vi "CyberSim.vi"() -> ()   [LabVIEW 2013]
doc: "Top-level VI to run one simulation of the iRobot and environment."
uses:
  CyberSim interface/Simulation Configuration.ctl
  autograder/feedbackMode.ctl
  shared/iRobot Sensor Display.ctl
  iRobot/Sensor/Accelerometer.ctl
panel:
  in  "check grade":bool
  out "sequence number":i32
  in  "home camera":bool
  in  "play":bool
  out "Simulator Display":refnum<vi>(3d-picture)
  out "simulation running":bool
  in  "exit":bool
  in  "start":bool
  in  "stop":bool
  in  "pause":bool
  out "iRobot Sensor Display":T1 {"Right Wheel (mm/s)" scale=-500.0..500.0; "Left Wheel (mm/s)" scale=-500.0..500.0}
  in  "Front Panel Tabs":T3(tab)=enum."Configuration"
  out "Statechart Diagram Display (supports LabVIEW Statecharts only)":picture
  out "Feedback":string
  in  "simulation configuration":T4={"maxTime"=inf, "enableVisualization"=TRUE, "statechart"=path "../src/LabVIEW/Statechart/Simulation Statechart.vi", "environment"=path "Environment - Navigation and Hill Climb 1.xml", "record"=path "Simulation Record.xml", "autograde?"=FALSE, "interactive?"=FALSE, "feedback mode"=enum."debug navigation"}
  in  "save configuration":bool
  in  "terminate at simulation end?":bool
  out "simulation time (s)":sgl format="%7.3g"
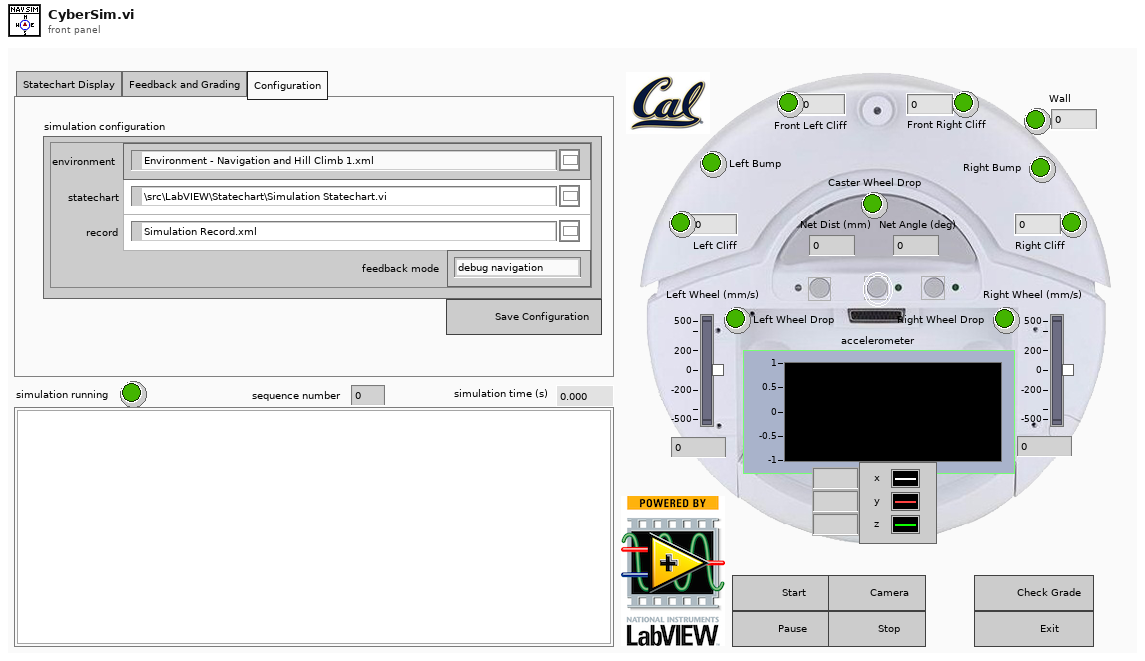
[diagram p1: front panel]
types:
  T1 = typedef "iRobot Sensor Display.ctl" = cluster{"Caster Wheel Drop":bool, "Left Wheel Drop":bool, "Right Wheel Drop":bool, "Left Bump":bool, "Right Bump":bool, "Left Cliff":bool, "Front Left Cliff":bool, "Front Right Cliff":bool, "Right Cliff":bool, "Wall":bool, "Net Dist (mm)":i32, "Net Angle (deg)":i32, "Wall":u16, "Left Cliff":u16, "Front Left Cliff":u16, "Front Right Cliff":u16, "Right Cliff":u16, "Left Wheel (mm/s)":i16, "Right Wheel (mm/s)":i16, "accelerometer":T2}
  T2 = typedef "Accelerometer.ctl" = cluster{"x axis (g)":dbl, "y axis (g)":dbl, "z axis (g)":dbl}
  T3 = enum32{"Statechart Display", "Feedback and Grading", "Configuration"}
  T4 = typedef "Simulation Configuration.ctl" = cluster{"maxTime":sgl, "enableVisualization":bool, "statechart":path, "environment":path, "record":path, "autograde?":bool, "interactive?":bool, "feedback mode":T5}
  T5 = typedef "feedbackMode.ctl" = enum32{"debug navigation", "debug hill climb", "autograde navigation", "autograde hill climb"}
  T6 = typedef "Simulator.ctl" = cluster{"configuration":T4, "Bump Sensors":refnum<k20>[], "Distance Sensors":refnum<k20>[], "Accelerometer":refnum<k20>, "Wall Sensor":refnum<k20>, "Statechart\ndisplay":refnum<vi>, "Body":refnum<k20>, "Left Motor":refnum<class "DC Motor Controller.lvclass">, "Right Motor":refnum<class "DC Motor Controller.lvclass">, "first step?":bool}
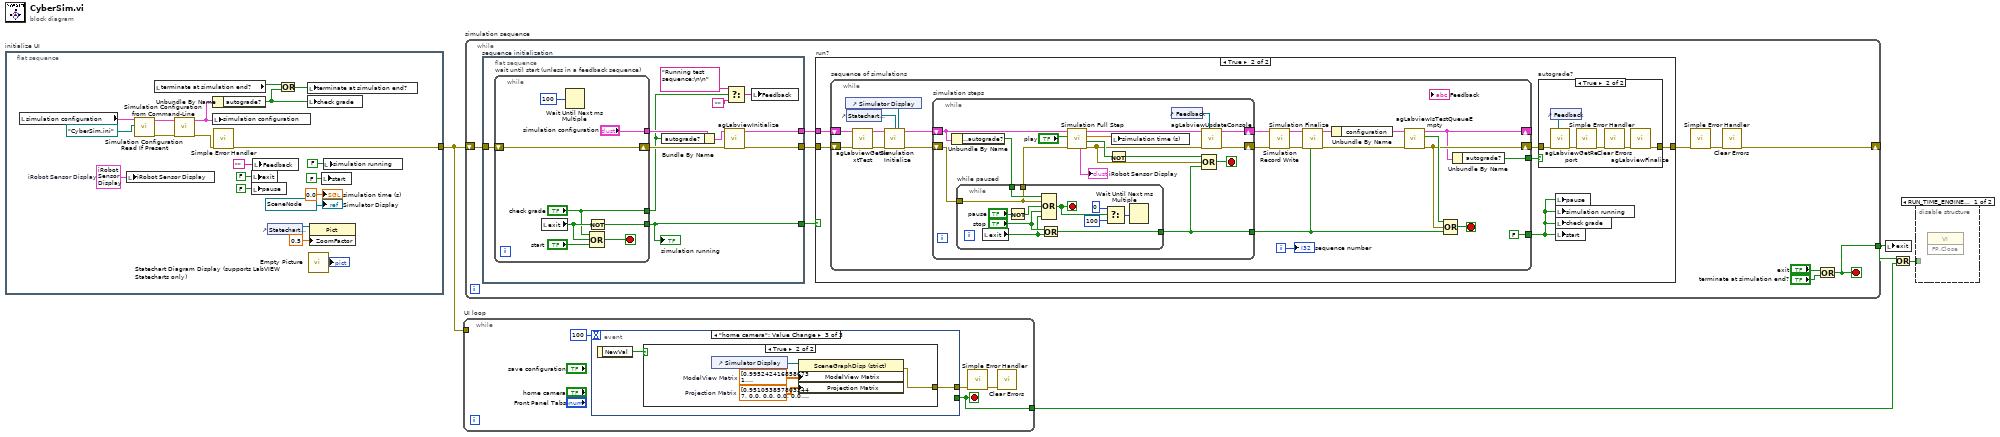
[diagram p0: block diagram]
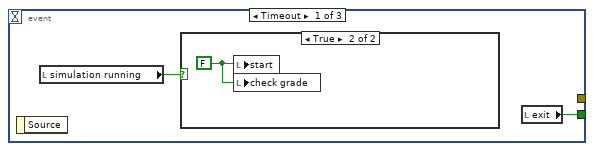
[diagram p3: hidden frame]
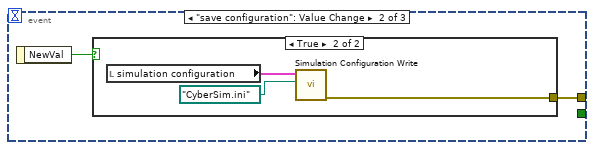
[diagram p5: hidden frame]
diagram:
  n1 = flat-sequence "initialize UI" {
    tunnel: [w21] -> w4
    frame #0 {
      w24 = T1 {"Caster Wheel Drop"=FALSE, "Left Wheel Drop"=FALSE, "Right Wheel Drop"=FALSE, "Left Bump"=FALSE, "Right Bump"=FALSE, "Left Cliff"=FALSE, "Front Left Cliff"=FALSE, "Front Right Cliff"=FALSE, "Right Cliff"=FALSE, "Wall"=FALSE, "Net Dist (mm)"=0, "Net Angle (deg)"=0, "Wall"=0, "Left Cliff"=0, "Front Left Cliff"=0, "Front Right Cliff"=0, "Right Cliff"=0, "Left Wheel (mm/s)"=0, "Right Wheel (mm/s)"=0, "accelerometer"={"x axis (g)"=0.0, "y axis (g)"=0.0, "z axis (g)"=0.0}}  # iRobot Sensor Display
      n2 = local read "simulation configuration"() -> (w19:T4)
      n3 = local write "iRobot Sensor Display"(w24) -> ()
      n4 = call "Simulation Configuration Read If Present.vi"("configuration"=path "CyberSim.ini", "simulation configuration"=w19) -> ("error out"=w17:errorcluster, "simulation configuration"=w18:T4)  [unwired: 8 in]
      n5 = local read "terminate at simulation end?"() -> (w9:bool)
      n6 = call "Simulation Configuration from Command-Line.vi"("error in"=w17, "simulation configuration in"=w18) -> ("error out"=w16:errorcluster, "simulation configuration out"=w14:T4)  [unwired: 8 in]
      n7 = Unbundle By Name(w14) -> ("autograde?"=w8:bool)
      n8 = local write "simulation configuration"(w14) -> ()
      n9 = call <vilib>:"Simple Error Handler.vi"("error in (no error)"=w16) -> ("error out"=w21:errorcluster)  [unwired: 4 in, 4 out]
      n10 = local write "exit"(FALSE ("exit")) -> ()
      n11 = local write "pause"(FALSE ("pause")) -> ()
      n12 = local write "Feedback"("") -> ()
      n13 = control-ref of="Statechart Diagram Display (supports LabVIEW Statecharts only)"() -> (w6:refnum<vi>)
      n14 = Or(x=w9, y=w8) -> (x .or. y?=w10:bool)
      n15 = local write "terminate at simulation end?"(w10) -> ()
      n16 = local write "check grade"(w8) -> ()
      n17 = call "Empty Picture"() -> ("empty picture"=→"Statechart Diagram Display (supports LabVIEW Statecharts only)":picture)
      n18 = property class="Pict"(reference=w6, "ZoomFactor"=sgl 0.5 ("Zoom Factor")) -> ()  [unwired: 1 in, 2 out]
      n19 = local write "start"(FALSE ("start")) -> ()
      n20 = local write "simulation running"(FALSE ("simulation running")) -> ()
      "simulation time (s)" <- sgl 0.0 ("simulated time (s)")
      "Simulator Display" <- refnum<vi> refnum ("3D Picture")
    }
  }
  n21 = while "UI loop" {
    tunnel: [w27] -> w2
    tunnel: w4 -> [_]
    stop <- w27 stop-if-true
    n22 = event shown="[2] \"home camera\": Value Change" {
      selector: _ -> [_ _ _]
      dyn-events: _ -> [_ _ _]
      timeout: 100 -> [_ _ _]
      tunnel: [_ w33 w38] -> w28
      tunnel: [w31 _ _] -> w27
      event Timeout {
        n23 = event-data() -> ()  [unwired: 1 in, 1 out]
        n24 = local read "simulation running"() -> (w30:bool)
        n25 = case shown="True" w30 {
          frame False {
          }
          frame True {
            w32 = FALSE ("AutoGrade")
            n26 = local write "start"(w32) -> ()
            n27 = local write "check grade"(w32) -> ()
          }
        }
        n28 = local read "exit"() -> (w31:bool)
      }
      event "save configuration": Value Change {
        n29 = event-data() -> ("NewVal"=w34:bool)  [unwired: 1 in]
        n30 = case shown="True" w34 {
          tunnel: [_ w36] -> w33
          frame False {
          }
          frame True {
            n31 = local read "simulation configuration"() -> (w37:T4)
            n32 = call "Simulation Configuration Write.vi"("configuration"=path "CyberSim.ini", "simulation configuration"=w37) -> ("error out"=w36:errorcluster)  [unwired: 9 in]
          }
        }
      }
      event "home camera": Value Change {
        n33 = event-data() -> ("NewVal"=w39:bool)  [unwired: 1 in]
        n34 = case shown="True" w39 {
          tunnel: [_ w40] -> w38
          frame False {
          }
          frame True {
            w41 = sgl[][] [[0.95105386, 0.0, 0.0, 0.0], [0.0, 2.4142137, 0.0, 0.0], [0.0, 0.0, -1.0002, -0.020002], [0.0, 0.0, -1.0, 0.0]]  # Projection Matrix
            w42 = sgl[][] [[0.9952424, -0.09162651, 0.033122927, -2.4552457], [0.010721975, 0.44090375, 0.8974903, -1.0543748], [-0.09683793, -0.8928653, 0.43978852, -0.9396557], [0.0, 0.0, 0.0, 1.0]]  # ModelView Matrix
            n35 = control-ref of="Simulator Display"() -> (w43:refnum<vi>)
            n36 = property class="SceneGraphDisp (strict)"(reference=w43, "ModelView Matrix"=w42, "Projection Matrix"=w41) -> (error out=w40:errorcluster)  [unwired: 1 in, 1 out]
          }
        }
      }
    }
    n37 = call <vilib>:"Simple Error Handler.vi"("error in (no error)"=w28) -> ("error out"=w26:errorcluster)  [unwired: 4 in, 4 out]
    n38 = call <vilib>:"Clear Errors.vi"("error in (no error)"=w26) -> ()  [unwired: 6 in, 1 out]
  }
  n39 = while "simulation sequence" {
    tunnel: [w50] -> w3
    shift-right: [w48] -> _
    shift-left: w4 -> [w44]
    stop <- w50 stop-if-true
    n40 = flat-sequence "sequence initialization" {
      tunnel: [w126] -> w49
      tunnel: [w127] -> w47
      tunnel: [w122] -> w46
      tunnel: w44 -> [w125]
      frame #0 {
        n41 = while "wait until start (unless in a feedback sequence)" {
          shift-right: [w132] -> w124
          shift-left: w125 -> [w132]
          tunnel: ["check grade"] -> w121
          tunnel: ["simulation configuration"] -> w123
          tunnel: [w129] -> w122
          stop <- w136 stop-if-true
          n42 = local read "exit"() -> (w135:bool)
          n43 = Wait Until Next ms Multiple(millisecond multiple=u32 100) -> ()  [unwired: 1 out]
          n44 = Not(x=w135) -> (.not. x?=w129:bool)
          n45 = Compound Arithmetic op=OR("check grade", w135, "start") -> (w136:bool)
        }
        "simulation running" <- w122
        n46 = Bundle By Name(cluster=w123, "autograde?"=w121) -> (w128:T4)
        n47 = call "agLabviewInitialize.vi"("Error In"=w124, "simulation configuration"=w128) -> ("Error Out"=w127:errorcluster, "simulation configuration"=w126:T4)  [unwired: 8 in]
        n48 = Select(t="Running test sequence:\n\n", s=w121, f="") -> (s? t:f=w119:string)
        n49 = local write "Feedback"(w119) -> ()
      }
    }
    n50 = case "run?" shown="True" w46 {
      tunnel: w49 -> [_ w60]
      tunnel: w47 -> [w54 w59]
      tunnel: [w54 w56] -> w45
      frame False {
      }
      frame True {
        n51 = while "sequence of simulations" {
          shift-right: [w78] -> w57
          shift-left: w59 -> [w73]
          shift-right: [w68] -> _
          shift-left: w60 -> [w72]
          tunnel: [w77] -> w58
          tunnel: [FALSE] -> w55
          i -> [w90]
          stop <- w89 stop-if-true
          n52 = control-ref of="Simulator Display"() -> (w84:refnum<vi>)
          n53 = control-ref of="Statechart Diagram Display (supports LabVIEW Statecharts only)"() -> (w86:refnum<vi>)
          n54 = call "agLabviewGetNextTest.vi"("Error In"=w73, "simulation configuration"=w72) -> ("Error Out"=w74:errorcluster, "simulation configuration"=w75:T4)  [unwired: 8 in]
          n55 = call "Simulation Initialize.vi"("simulation configuration"=w75, "Statechart display"=w86, "Simulator display"=w84, "Error In"=w74) -> ("simulator"=w88:T6, "Error Out"=w87:errorcluster)  [unwired: 10 in]
          n56 = while "simulation steps" {
            shift-right: [w93] -> w83
            shift-left: w88 -> [w99]
            shift-right: [w92] -> w85
            shift-left: w87 -> [w97]
            tunnel: [w100] -> w79
            stop <- w104 stop-if-true
            n57 = Unbundle By Name(w99) -> ("configuration.autograde?"=w98:bool)
            n58 = while "while paused" {
              tunnel: [w113] -> w100
              tunnel: w97 -> [w107]
              tunnel: w98 -> [w108]
              tunnel: [w107] -> w96
              stop <- w109 stop-if-true
              n59 = local read "exit"() -> (w114:bool)
              n60 = Not(x="pause") -> (.not. x?=w116:bool)
              n61 = Or(x="stop", y=w114) -> (x .or. y?=w113:bool)
              n62 = Compound Arithmetic op=OR(w108, w107, w116, "stop", w114) -> (w109:bool)
              n63 = Select(t=u32 0 ("millisecond multiple"), s=w109, f=u32 100 ("millisecond multiple")) -> (s? t:f=w112:u32)
              n64 = Wait Until Next ms Multiple(millisecond multiple=w112) -> ()  [unwired: 1 out]
            }
            n65 = call "Simulation Full Step.vi"("Error In"=w96, "iRobot Play Button (false)"="play", "simulator"=w99) -> ("Error Out"=w95:errorcluster, "continue to next step?"=w105:bool, "simulated time (s)"=w102:sgl, "simulator"=w94:T6, "iRobot Sensor Display"=→"iRobot Sensor Display":T1)  [unwired: 4 in]
            n66 = Not(x=w105) -> (.not. x?=w101:bool)
            n67 = local write "simulation time (s)"(w102) -> ()
            n68 = control-ref of="Feedback"() -> (w91:refnum<vi>)
            n69 = call "agLabviewUpdateConsole.vi"("console"=w91, "Error In"=w95, "simulator"=w94) -> ("Error Out"=w92:errorcluster, "simulator"=w93:T6)  [unwired: 7 in]
            n70 = Compound Arithmetic op=OR(w101, w95, w100) -> (w104:bool)
          }
          n71 = call "Simulation Record Write.vi"("Error In"=w85, "simulator"=w83) -> ("Error Out"=w81:errorcluster, "simulator"=w82:T6)  [unwired: 8 in]
          n72 = call "Simulation Finalize.vi"("terminated by user?"=w79, "error in (no error)"=w81, "simulator"=w82) -> ("error out"=w70:errorcluster, "simulator"=w71:T6)  [unwired: 7 in]
          n73 = Unbundle By Name(w71) -> ("configuration"=w69:T4)
          n74 = call "agLabviewIsTestQueueEmpty.vi"("Error In"=w70, "simulation configuration"=w69) -> ("Error Out"=w78:errorcluster, "Empty?"=w80:bool, "simulation configuration"=w68:T4)  [unwired: 7 in]
          n75 = Compound Arithmetic op=OR(w80, w78, w79) -> (w89:bool)
          n76 = Unbundle By Name(w68) -> ("autograde?"=w77:bool)
          "sequence number" <- w90
        }
        n77 = case "autograde?" shown="True" w58 {
          tunnel: [w61 w67] -> w56
          tunnel: w57 -> [w61 w66]
          frame False {
          }
          frame True {
            n78 = control-ref of="Feedback"() -> (w65:refnum<vi>)
            n79 = call "agLabviewGetReport.vi"("console"=w65, "Error In"=w66) -> ("Error Out"=w63:errorcluster)  [unwired: 9 in]
            n80 = call <vilib>:"Simple Error Handler.vi"("error in (no error)"=w63) -> ("error out"=w64:errorcluster)  [unwired: 4 in, 4 out]
            n81 = call <vilib>:"Clear Errors.vi"("error in (no error)"=w64) -> ("error out"=w62:errorcluster)  [unwired: 6 in]
            n82 = call "agLabviewFinalize.vi"("Error In"=w62) -> ("Error Out"=w67:errorcluster)  [unwired: 10 in]
          }
        }
        n83 = local write "pause"(w55) -> ()
        n84 = local write "simulation running"(w55) -> ()
        n85 = local write "check grade"(w55) -> ()
        n86 = local write "start"(w55) -> ()
      }
    }
    n87 = call <vilib>:"Simple Error Handler.vi"("error in (no error)"=w45) -> ("error out"=w53:errorcluster)  [unwired: 4 in, 4 out]
    n88 = call <vilib>:"Clear Errors.vi"("error in (no error)"=w53) -> ("error out"=w48:errorcluster)  [unwired: 6 in]
    n89 = Or(x="exit", y="terminate at simulation end?") -> (x .or. y?=w50:bool)
  }
  n90 = local write "exit"(w3) -> ()
  n91 = Or(x=w3, y=w2) -> (x .or. y?=w1:bool)
  n92 = disable-structure shown="RUN_TIME_ENGINE==True" {
    disable-tunnel: w1 -> [_ _]
    frame condition #0 {
      n93 = invoke class="VI" method="FP.Close"() -> ()  [unwired: 3 in, 3 out]
    }
    frame condition #1 (active) {
    }
  }
